vi "Add Controls in Results.vi"(0 "Result Cluster":refnum<vi>, 1 "Output Clusters in":string[](array[string]), 5 "VI Reference":refnum<vi>, 7 "Ctl Refnum":refnum<vi>, 11 "error in":errorcluster) -> (4 "Output Clusters out":string[](array[string]), 15 "error out":errorcluster)   [LabVIEW 2021, in "Converter.lvlib"]
uses:
  Converter.lvlib
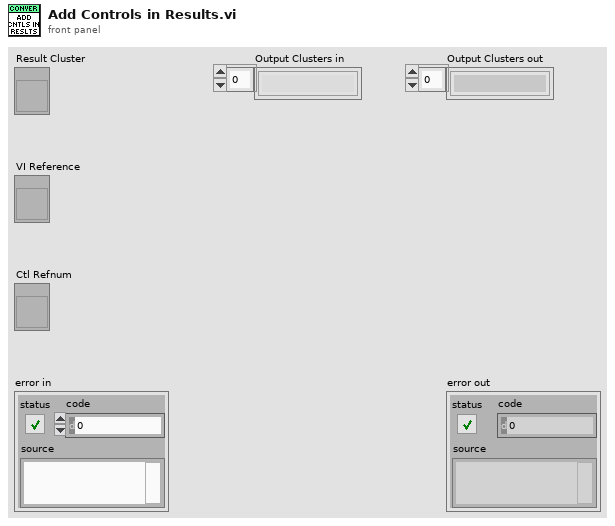
[diagram p1: front panel]
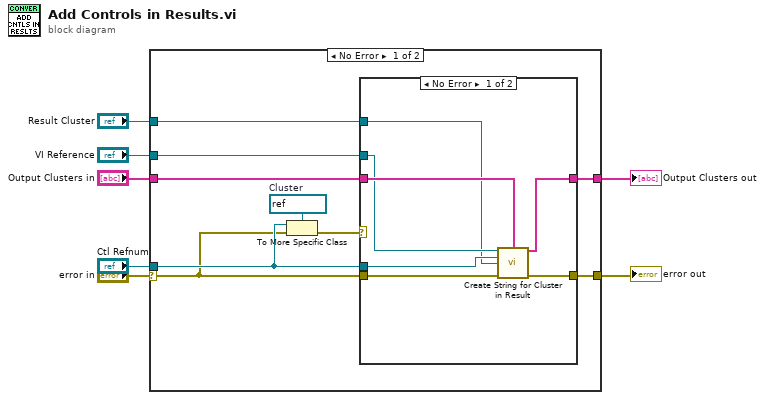
[diagram p0: block diagram]
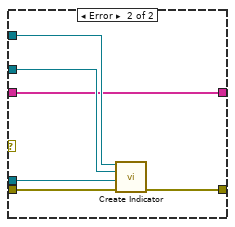
[diagram p2: hidden frame]
diagram:
  n1 = case shown="No Error" "error in" {
    selector: "error in" -> [w8 w30]
    tunnel: "Output Clusters in" -> [w16 _]
    tunnel: [w15 _] -> w6
    tunnel: "Ctl Refnum" -> [w14 _]
    tunnel: "VI Reference" -> [w11 _]
    tunnel: [w10 w30] -> w3
    tunnel: "Result Cluster" -> [w9 _]
    frame No Error {
      w12 = refnum<vi> refnum  # Cluster
      n2 = To More Specific Class(target class=w12, reference=w14, error in=w8) -> (error out=w13:errorcluster)  [unwired: 1 out]
      n3 = case shown="No Error" w13 {
        tunnel: w9 -> [w18 w29]
        tunnel: [w17 w28] -> w10
        tunnel: w11 -> [w20 w27]
        tunnel: w14 -> [w19 w26]
        tunnel: w8 -> [w23 w25]
        tunnel: [w22 w24] -> w15
        tunnel: w16 -> [w21 w24]
        frame No Error {
          n4 = call "Create String for Cluster in Result.vi"("VI Reference"=w20, "Output CLuster[]"=w21, "Ctl Refnum"=w19, "Result Cluster"=w18, "error in (no error)"=w23) -> ("Output Clusters"=w22:string[], "error out"=w17:errorcluster)  [unwired: 9 in]
        }
        frame Error {
          n5 = call "Create Indicator.vi"("Result Cluster"=w29, "VI Reference"=w27, "Ctl Refnum"=w26, "error in (no error)"=w25) -> ("error out"=w28:errorcluster)  [unwired: 11 in]
        }
      }
    }
    frame Error {
    }
  }
  "Output Clusters out" <- w6
  "error out" <- w3
